vi "ExpiredError.vi"(7 "Timeout":u32, 8 "error in (no error)":errorcluster, 10 "Watchdog Name":string, 11 "Expired":bool) -> (0 "error out":errorcluster)   [LabVIEW 2017, in "Pound.lvclass"]
uses:
  <vilib>/NI/Software Watchdog/Pound/Pound.lvclass
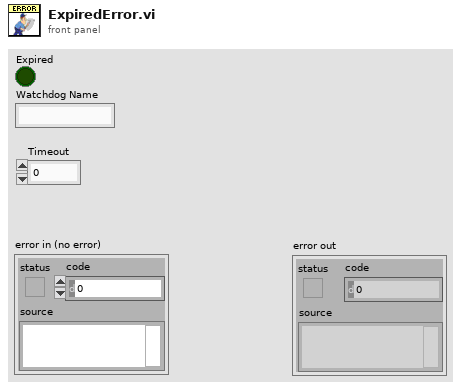
[diagram p1: front panel]
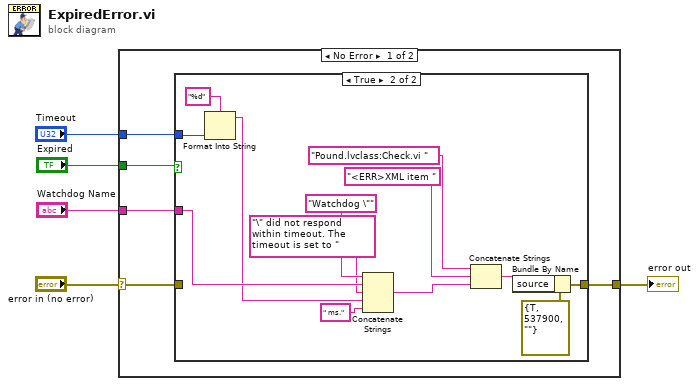
[diagram p0: block diagram]
diagram:
  n1 = case shown="No Error" "error in (no error)" {
    selector: "error in (no error)" -> [w8 w25]
    tunnel: [w7 w25] -> w4
    tunnel: "Expired" -> [w10 _]
    tunnel: "Watchdog Name" -> [w9 _]
    tunnel: "Timeout" -> [w6 _]
    frame No Error {
      n2 = case shown="True" w10 {
        tunnel: w9 -> [_ w23]
        tunnel: w8 -> [w11 _]
        tunnel: [w11 w16] -> w7
        tunnel: w6 -> [_ w15]
        frame False {
        }
        frame True {
          n3 = Format Into String(format string="%d", w15) -> (resulting string=w13:string)  [unwired: 2 in, 1 out]
          n4 = Concatenate Strings("Watchdog \"", w23, "\" did not respond within timeout. The timeout is set to ", w13, " ms." ("string")) -> (w17:string)
          n5 = Concatenate Strings("Pound.lvclass:Check.vi " ("string"), "<ERR>XML item " ("Format String"), w17) -> (w19:string)
          n6 = Bundle By Name(cluster=errorcluster {"status"=TRUE, "code"=537900, "source"=""} ("error in"), "source"=w19) -> (w16:errorcluster)
        }
      }
    }
    frame Error {
    }
  }
  "error out" <- w4
